vi "Limit.vi"(9 "MeasuredFreq":dbl=63.99936700000001 format="%#_12f", 10 "TLcu":dbl=21.0 format="%#_12f", 11 "OkFreq":dbl=64.0 format="%0#_12f") -> (2 "MeasureFreq_max":dbl format="%#_12f", 3 "MeasureFreq_min":dbl format="%#_12f")   [LabVIEW 2009]
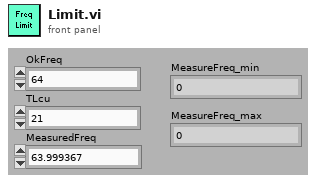
[diagram p1: front panel]
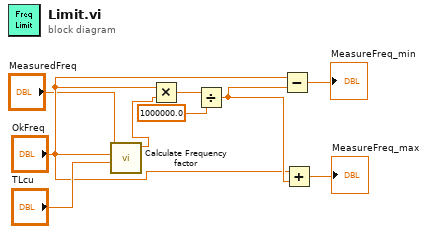
[diagram p0: block diagram]
diagram:
  n1 = call "Calculate Frequency factor.vi"("TLcu"="TLcu", "OkFreq"="OkFreq", "MeasuredFreq"="MeasuredFreq") -> ("PPM"=w1:dbl)  [unwired: 1 in, 7 out]
  n2 = Multiply(x="OkFreq", y=w1) -> (x*y=w8:dbl)
  n3 = Divide(x=w8, y=1000000.0) -> (x/y=w6:dbl)
  n4 = Subtract(x="OkFreq", y=w6) -> (x-y=→"MeasureFreq_min":dbl)
  n5 = Add(x="OkFreq", y=w6) -> (x+y=→"MeasureFreq_max":dbl)
